vi "PathPlanner_DriveFeedFwds_Reverse.vi"(11 "in DriveFeedFwds":T1) -> (0 "Error":bool, 3 "reverse DriveFeedFwds":T1)   [LabVIEW 2019, in "PathPlanner24.lvlib"]
doc: "Interpolate between this state and the given state\n \nInputs: \n - trajectoryState - cluster - this trajectory state\n - endVal - cluster - State to interpolate with\n - t - double - Interpolation factor (0.0-1.0)\n\nOutputs:\n - Interpolated state - trajectory state - interpolated state"
uses:
  TypeDef/PathPlannerDriveFeedFwds.ctl
  PathPlanner_FieldUtil_SymmetryType.vi
  PathPlanner24.lvlib
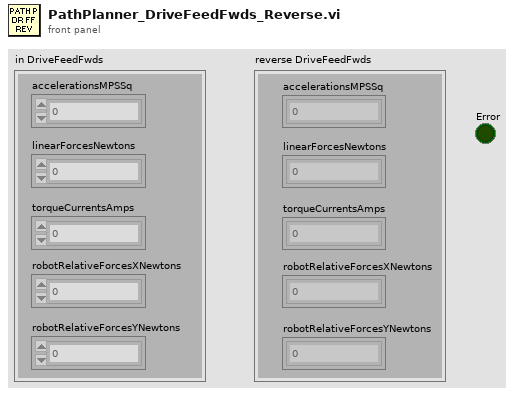
[diagram p1: front panel]
types:
  T1 = typedef "PathPlanner24.lvlib/PathPlannerDriveFeedFwds.ctl" = cluster{"accelerationsMPSSq":dbl[], "linearForcesNewtons":dbl[], "torqueCurrentsAmps":dbl[], "robotRelativeForcesXNewtons":dbl[], "robotRelativeForcesYNewtons":dbl[]}
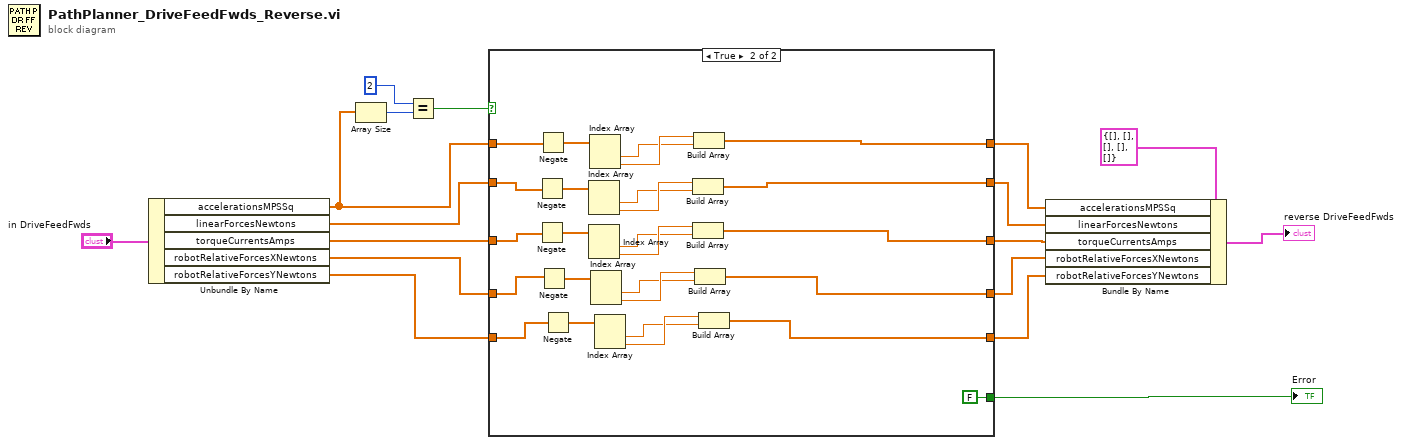
[diagram p0: block diagram]
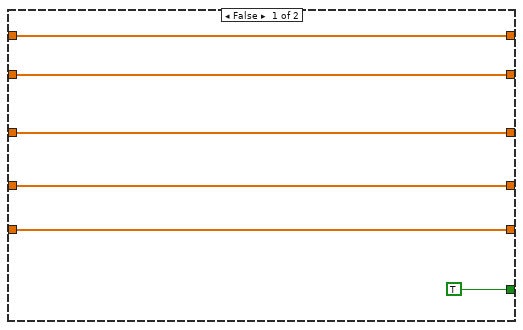
[diagram p2: hidden frame]
diagram:
  n1 = Unbundle By Name("in DriveFeedFwds") -> ("accelerationsMPSSq"=w11:dbl[], "linearForcesNewtons"=w10:dbl[], "torqueCurrentsAmps"=w9:dbl[], "robotRelativeForcesXNewtons"=w8:dbl[], "robotRelativeForcesYNewtons"=w7:dbl[])
  n2 = Array Size(array=w11) -> (size(s)=w14:i32)
  n3 = Equal?(x=2, y=w14) -> (x = y?=w12:bool)
  n4 = case shown="True" w12 {
    tunnel: w11 -> [w22 w49]
    tunnel: w10 -> [w21 w33]
    tunnel: w9 -> [w20 w32]
    tunnel: w8 -> [w19 w31]
    tunnel: w7 -> [w18 w30]
    tunnel: [TRUE FALSE] -> w6
    tunnel: [w22 w29] -> w5
    tunnel: [w21 w28] -> w4
    tunnel: [w20 w27] -> w3
    tunnel: [w19 w26] -> w2
    tunnel: [w18 w25] -> w1
    frame False {
    }
    frame True {
      n5 = Negate(x=w33) -> (-x=w45:dbl[])
      n6 = Negate(x=w32) -> (-x=w42:dbl[])
      n7 = Negate(x=w49) -> (-x=w48:dbl[])
      n8 = Negate(x=w31) -> (-x=w39:dbl[])
      n9 = Negate(x=w30) -> (-x=w36:dbl[])
      n10 = Index Array(array=w45) -> (element #1=w43:dbl, element #2=w44:dbl)  [unwired: 2 in]
      n11 = Index Array(array=w42) -> (element #1=w40:dbl, element #2=w41:dbl)  [unwired: 2 in]
      n12 = Index Array(array=w48) -> (element #1=w46:dbl, element #2=w47:dbl)  [unwired: 2 in]
      n13 = Index Array(array=w39) -> (element #1=w37:dbl, element #2=w38:dbl)  [unwired: 2 in]
      n14 = Index Array(array=w36) -> (element #1=w34:dbl, element #2=w35:dbl)  [unwired: 2 in]
      n15 = Build Array(w44, w43) -> (w28:dbl[])
      n16 = Build Array(w41, w40) -> (w27:dbl[])
      n17 = Build Array(w47, w46) -> (w29:dbl[])
      n18 = Build Array(w38, w37) -> (w26:dbl[])
      n19 = Build Array(w35, w34) -> (w25:dbl[])
    }
  }
  "Error" <- w6
  n20 = Bundle By Name(cluster=T1 {"accelerationsMPSSq"=[], "linearForcesNewtons"=[], "torqueCurrentsAmps"=[], "robotRelativeForcesXNewtons"=[], "robotRelativeForcesYNewtons"=[]} ("PathPlannerState"), "accelerationsMPSSq"=w5, "linearForcesNewtons"=w4, "torqueCurrentsAmps"=w3, "robotRelativeForcesXNewtons"=w2, "robotRelativeForcesYNewtons"=w1) -> (→"reverse DriveFeedFwds":T1)
